vi "GetWaveformByBusName.vi"(8 "error in (no error)":errorcluster, 10 "Bus Name":string, 11 "Acq Waveforms":waveform(sgl)[](array[waveform])) -> (0 "error out":errorcluster, 2 "Waveform in ABC Order":waveform(dbl)[](array[waveform]), 3 "Acq Waveforms Out":waveform(sgl)[](array[waveform]))   [LabVIEW 2017, in "McsaUtilities.lvlib"]
uses:
  <vilib>/addons/InsightCM/Utilities/MCSA/McsaUtilities.lvlib
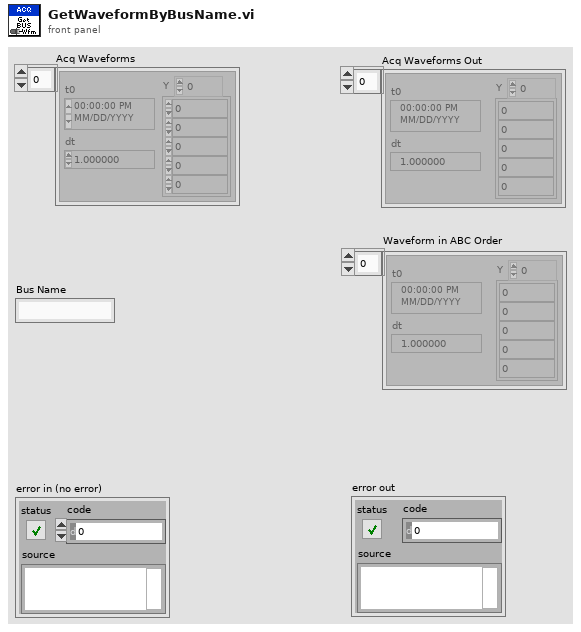
[diagram p1: front panel]
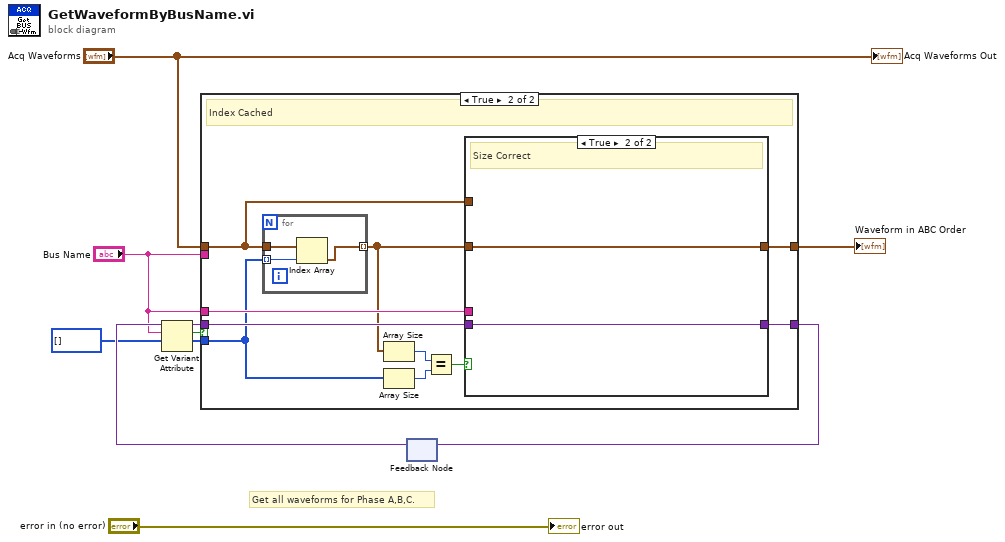
[diagram p0: block diagram]
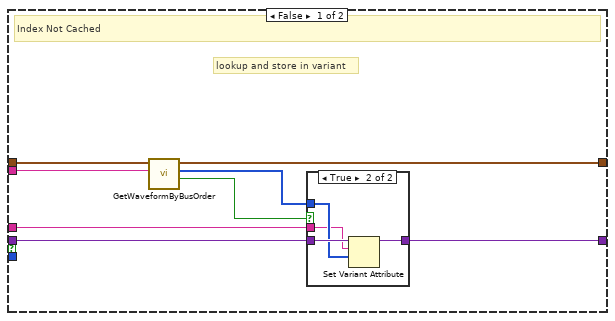
[diagram p2: hidden frame]
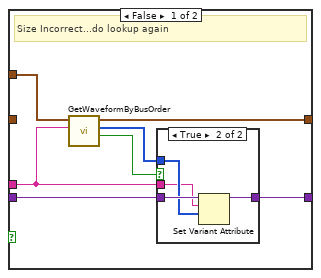
[diagram p4: hidden frame]
diagram:
  # "Get all waveforms for Phase A,B,C."
  n1 = feedback #1() -> (w5:variant)  [unwired: 1 in]
  n2 = Get Variant Attribute(Variant=w5, name="Bus Name", default value (empty Variant)=i32[] []) -> (duplicate Variant=w7:variant, found=w6:bool, value=w8:i32[])  [unwired: 1 in, 1 out]
  n3 = case shown="True" w6 {
    tunnel: [w11 w30] -> w2
    tunnel: "Acq Waveforms" -> [w15 w29]
    tunnel: "Bus Name" -> [w14 _]
    tunnel: w7 -> [w18 w33]
    tunnel: w8 -> [_ w27]
    tunnel: "Bus Name" -> [w17 w31]
    tunnel: [w16 w32] -> w9
    frame False {
      # "lookup and store in variant"
      # "Index Not Cached"
      n4 = call <vilib>:"GetWaveformByBusOrder.vi"("Bus Name"=w14, "Acq Waveforms"=w15) -> ("found?"=w12:bool, "Index in ABC order"=w13:i32[], "Bus Waveforms in ABC order"=w11:waveform(dbl)[])  [unwired: 7 in]
      n5 = case shown="True" w12 {
        tunnel: w13 -> [_ w22]
        tunnel: w18 -> [w19 w23]
        tunnel: w17 -> [_ w21]
        tunnel: [w19 w20] -> w16
        frame False {
        }
        frame True {
          n6 = Set Variant Attribute(Variant=w23, name=w21, value=w22) -> (Variant out=w20:variant)  [unwired: 1 in, 2 out]
        }
      }
    }
    frame True {
      # "Index Cached"
      n7 = for {
        tunnel: w29 -> [w36]
        tunnel: w27 -> [w35] mode=indexing
        tunnel: [w34] -> w28 mode=indexing
        n8 = Index Array(array=w36, index=w35) -> (element=w34:waveform(sgl))
      }
      n9 = Array Size(array=w28) -> (size(s)=w26:i32)
      n10 = Array Size(array=w27) -> (size(s)=w25:i32)
      n11 = Equal?(x=w26, y=w25) -> (x = y?=w24:bool)
      n12 = case shown="True" w24 {
        tunnel: [w40 w49] -> w30
        tunnel: [w42 w50] -> w32
        tunnel: w33 -> [w43 w50]
        tunnel: w31 -> [w37 _]
        tunnel: w29 -> [w41 _]
        tunnel: w28 -> [_ w49]
        frame False {
          # "Size Incorrect...do lookup again"
          n13 = call <vilib>:"GetWaveformByBusOrder.vi"("Bus Name"=w37, "Acq Waveforms"=w41) -> ("found?"=w39:bool, "Index in ABC order"=w38:i32[], "Bus Waveforms in ABC order"=w40:waveform(dbl)[])  [unwired: 7 in]
          n14 = case shown="True" w39 {
            tunnel: w38 -> [_ w47]
            tunnel: w43 -> [w44 w48]
            tunnel: w37 -> [_ w46]
            tunnel: [w44 w45] -> w42
            frame False {
            }
            frame True {
              n15 = Set Variant Attribute(Variant=w48, name=w46, value=w47) -> (Variant out=w45:variant)  [unwired: 1 in, 2 out]
            }
          }
        }
        frame True {
          # "Size Correct"
        }
      }
    }
  }
  "Waveform in ABC Order" <- w2
  n16 = feedback-in #1(w9) -> ()
  "Acq Waveforms Out" <- "Acq Waveforms"
  "error out" <- "error in (no error)"
